vi "GUI - Multi TDMS Files Preview.vi"(5 "error in (no error)":errorcluster, 6 "ReInit All to Default?":bool, 7 "Application Name":string="GenUtil", 9 "State Queue":T1[](array[typedef])=["SC >>> Initialize"]) -> (19 "error out":errorcluster)   [LabVIEW 2020, in "TDMS.lvclass"]
uses:
  TDMS.lvclass
  API/Generic Utilities_class/utils/GenUtil State List.ctl
  <vilib>/Utility/sysdir.llb/System Directory Type.ctl
  <vilib>/Platform/browser.llb/Open URL in Default Browser (path).vi
  API/Generic Utilities_class/Generic Utilities.lvclass
  <vilib>/addons/_AddQ/G#Object/G#Object.lvclass
panel:
  in  "Task":enum32{"Monitor", "Settings"}(tab)
  in  "Select TDMS File":path
  out "group/channel names":string[][](array[string])
  out "value":variant
  out "found":bool
  in  "AppData Folder":bool
  out "State History":string[](array[string])
  out "State Index":i32
  in  "State 1":bool
  in  "Exit":bool
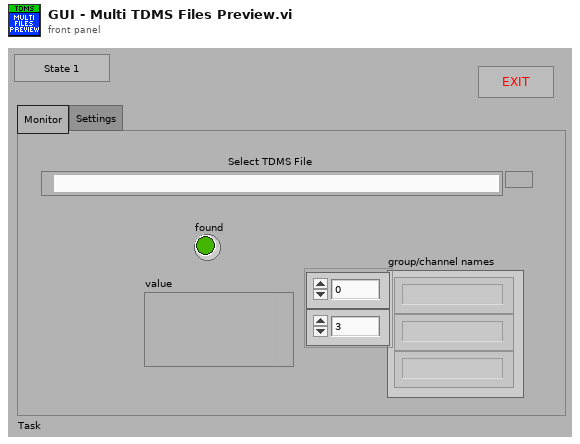
[diagram p1: front panel]
types:
  T1 = typedef "Generic Utilities.lvclass/GenUtil State List.ctl" = string
  T2 = enum32{"Invalid", "Standard", "Closed", "Hidden", "Minimized", "Maximized"}
  T3 = typedef "System Directory Type.ctl" = i32
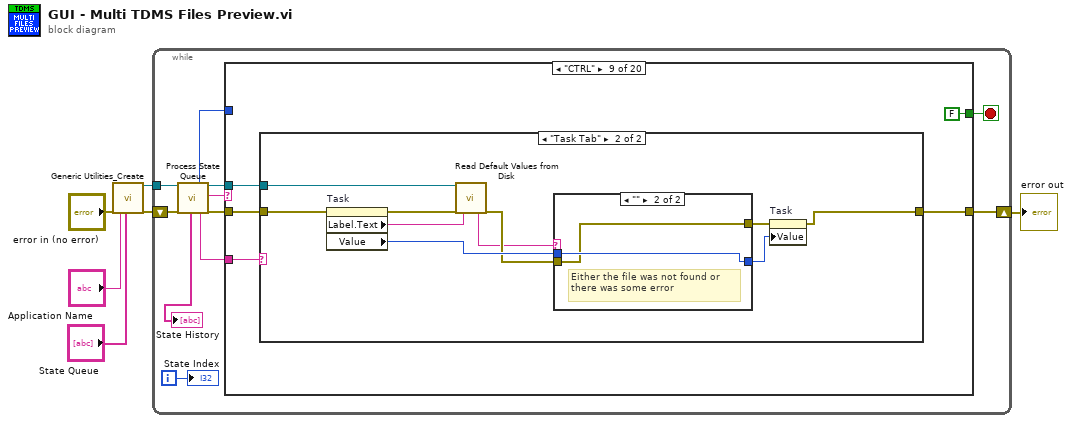
[diagram p0: block diagram]
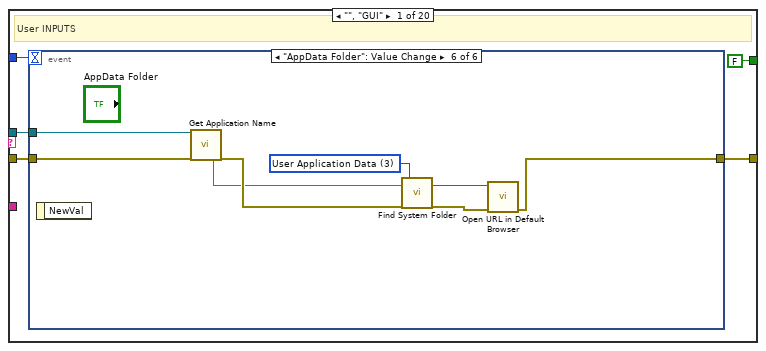
[diagram p2: hidden frame]
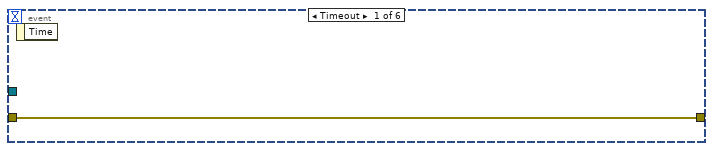
[diagram p3: hidden frame]
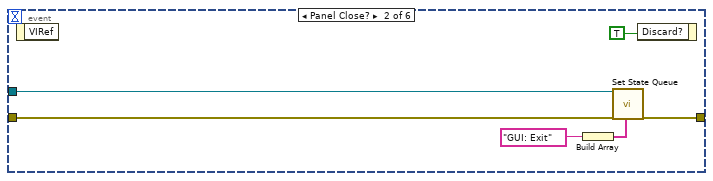
[diagram p4: hidden frame]
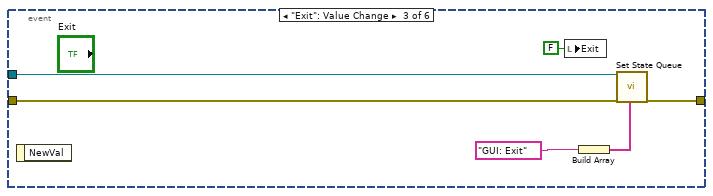
[diagram p5: hidden frame]
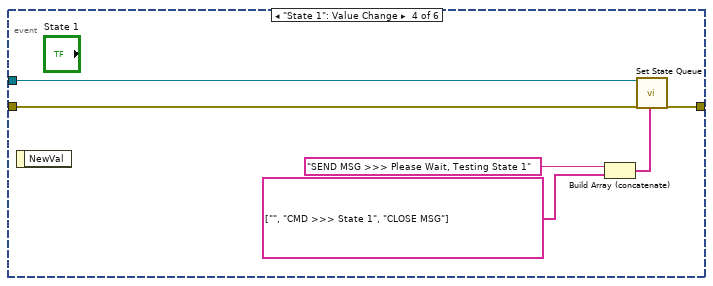
[diagram p6: hidden frame]
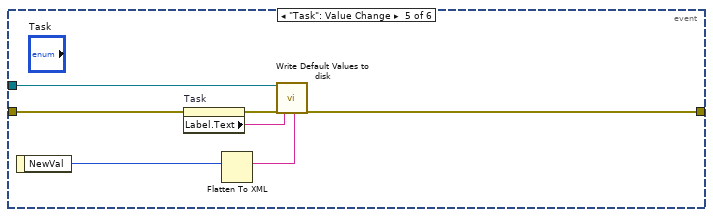
[diagram p7: hidden frame]
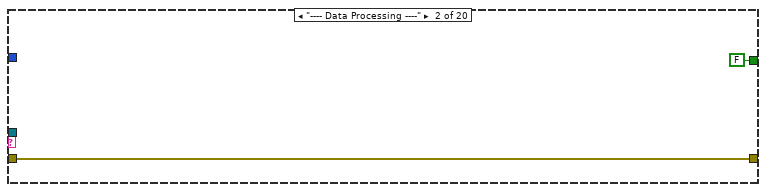
[diagram p8: hidden frame]
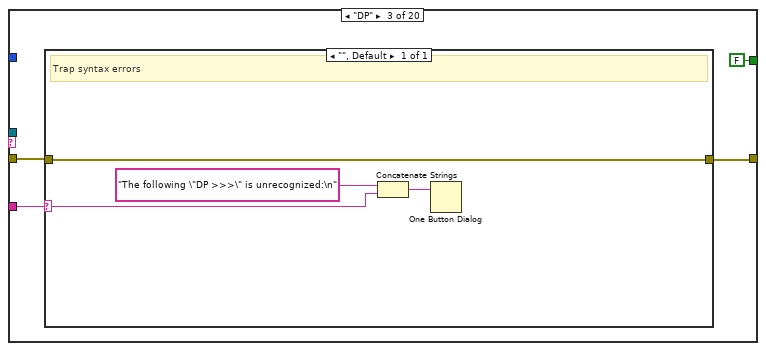
[diagram p9: hidden frame]
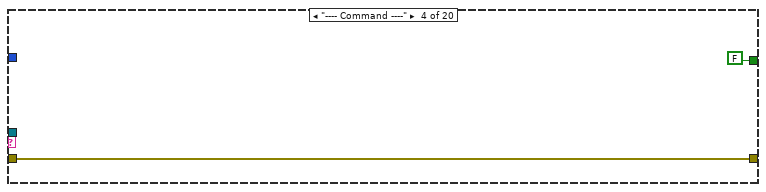
[diagram p10: hidden frame]
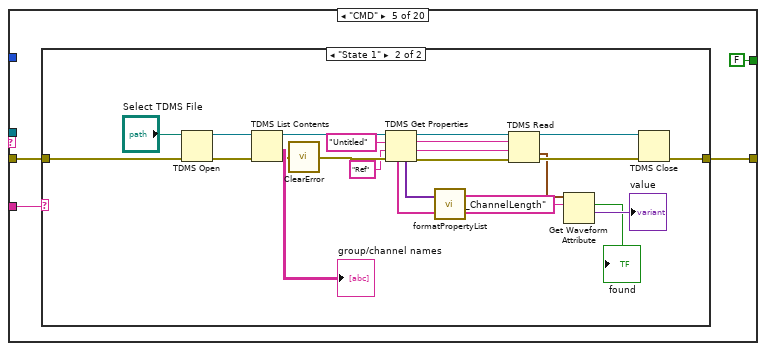
[diagram p11: hidden frame]
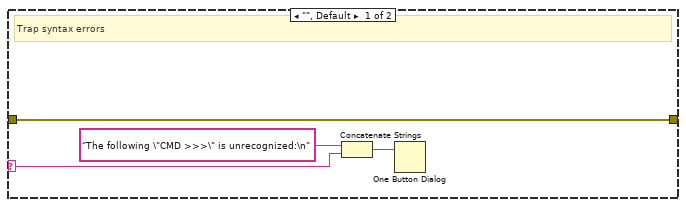
[diagram p12: hidden frame]
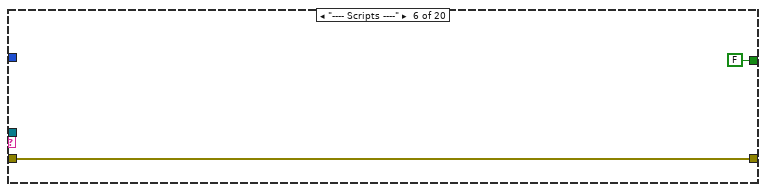
[diagram p13: hidden frame]
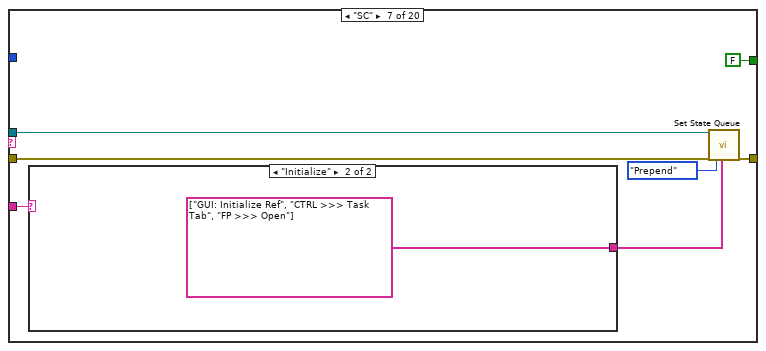
[diagram p14: hidden frame]
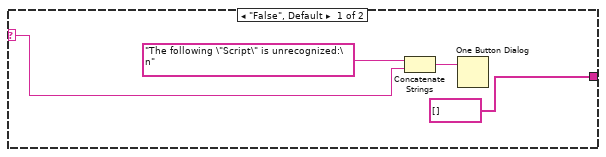
[diagram p15: hidden frame]
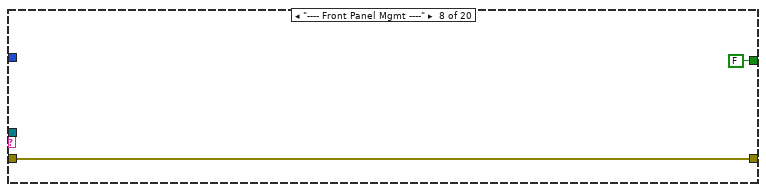
[diagram p16: hidden frame]
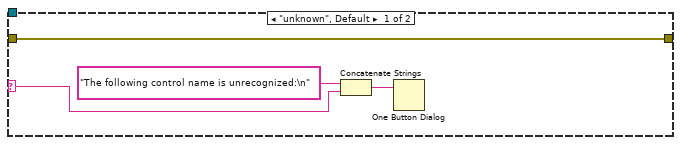
[diagram p17: hidden frame]
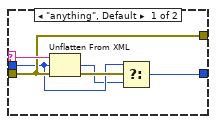
[diagram p18: hidden frame]
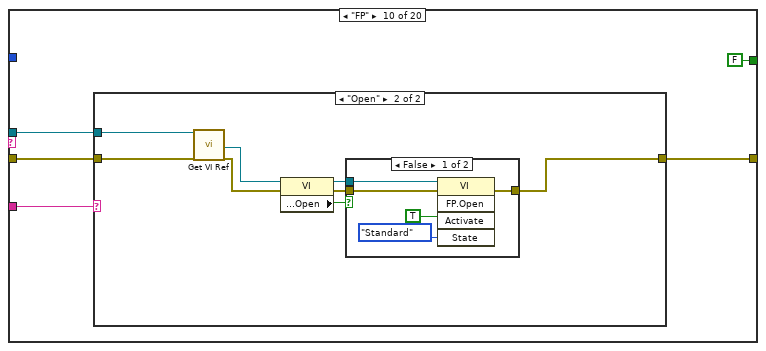
[diagram p19: hidden frame]
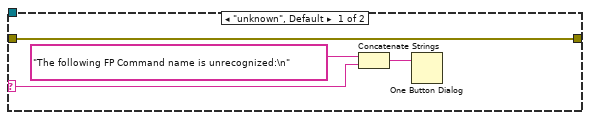
[diagram p20: hidden frame]
diagram:
  n1 = call "Generic Utilities_Create.vi"("error in (no error)"="error in (no error)", "Application Name"="Application Name", "State Queue"="State Queue") -> ("reference out"=w6:refnum<class "Generic Utilities.lvclass">, "error out"=w5:errorcluster)  [unwired: 15 in]
  n2 = while {
    shift-right: [w9] -> w1
    shift-left: w5 -> [w14]
    tunnel: w6 -> [w15]
    i -> [w16]
    stop <- w17 stop-if-true
    n3 = call "Process State Queue.vi"("reference in"=w15, "error in (no error)"=w14) -> ("State History"=→"State History":string[], "Timeout"=w13:i32, "State Option"=w8:string, "reference out"=w12:refnum<class "Generic Utilities.lvclass">, "Current State"=w11:string, "error out"=w10:errorcluster)  [unwired: 10 in, 2 out]
    n4 = case shown="\"CTRL\"" w11 {
      selector: w11 -> [_ _ _ _ _ _ _ _ _ _ _ _ _ _ _ _ w266 _ _ _]
      tunnel: w12 -> [w20 _ _ _ _ _ w107 _ w118 w146 _ w176 w189 w225 w250 _ _ _ _ w276]
      tunnel: [FALSE FALSE FALSE FALSE FALSE FALSE FALSE FALSE FALSE FALSE FALSE FALSE TRUE FALSE FALSE FALSE FALSE FALSE FALSE TRUE] -> w17
      tunnel: w13 -> [w21 _ _ _ _ _ _ _ _ _ _ _ _ _ _ _ _ _ _ _]
      tunnel: w8 -> [_ _ w61 _ w71 _ w103 _ w119 w143 _ _ _ w234 _ _ _ _ _ _]
      tunnel: w10 -> [w19 w57 w60 w67 w69 w100 w106 w114 w116 w145 w166 w172 w186 w224 w251 w262 w264 w269 w272 w275]
      tunnel: [w18 w57 w59 w67 w70 w100 w105 w114 w117 w144 w166 w173 w185 w222 w247 w262 w264 errorcluster {"status"=FALSE, "code"=0, "source"=""} ("error out") w272 w274] -> w9
      frame "", "GUI" {
        # "User INPUTS"
        n5 = event shown="[5] \"AppData Folder\": Value Change" {
          selector: _ -> [_ _ _ _ _ _]
          dyn-events: _ -> [_ _ _ _ _ _]
          timeout: w21 -> [_ _ _ _ _ _]
          tunnel: w20 -> [_ w28 w34 w40 w47 w55]
          tunnel: w19 -> [w23 w27 w32 w39 w44 w54]
          tunnel: [w23 w26 w33 w41 w42 w49] -> w18
          event Timeout {
            n6 = event-data() -> ()  [unwired: 1 in, 1 out]
          }
          event Panel Close? {
            n7 = event-data() -> ()  [unwired: 1 in, 1 out]
            n8 = Build Array(T1 "GUI: Exit" ("State List")) -> (w25:T1[])
            n9 = call "Set State Queue.vi"("reference in"=w28, "error in (no error)"=w27, "State Queue"=w25) -> ("error out"=w26:errorcluster)  [unwired: 15 in, 1 out]
            n10 = event-data("Discard?"=TRUE) -> ()  [unwired: 1 in, 1 out]
          }
          event "Exit": Value Change {
            n11 = event-data() -> ()  [unwired: 1 in, 1 out]
            n12 = local write "Exit"(FALSE ("Exit")) -> ()
            n13 = Build Array(T1 "GUI: Exit" ("State List")) -> (w31:T1[])
            n14 = call "Set State Queue.vi"("reference in"=w34, "error in (no error)"=w32, "State Queue"=w31) -> ("error out"=w33:errorcluster)  [unwired: 15 in, 1 out]
          }
          event "State 1": Value Change {
            n15 = event-data() -> ()  [unwired: 1 in, 1 out]
            n16 = Build Array (concatenate)("SEND MSG >>> Please Wait, Testing State 1" ("String"), T1[] ["", "CMD >>> State 1", "CLOSE MSG"] ("State Queue OUT")) -> (w36:T1[])
            n17 = call "Set State Queue.vi"("reference in"=w40, "error in (no error)"=w39, "State Queue"=w36) -> ("error out"=w41:errorcluster)  [unwired: 15 in, 1 out]
          }
          event "Task": Value Change {
            n18 = event-data() -> ("NewVal"=w48:enum32{"Monitor", "Settings"})  [unwired: 1 in]
            n19 = property on="Task" class="TabCtl (strict)"(error in=w44) -> (error out=w43:errorcluster, "Label.Text"=w46:string)  [unwired: 1 in, 1 out]
            n20 = Flatten To XML(6:w48) -> (2:w45:string)
            n21 = call-dynamic "Write Default Values to disk.vi"("reference in"=w47, "error in (no error)"=w43, "Control Label"=w46, "Value (XML String)"=w45) -> ("error out"=w42:errorcluster)  [unwired: 14 in, 1 out]
          }
          event "AppData Folder": Value Change {
            w56 = T3 3 items=["User Home"=0, "User Desktop"=1, "User Documents"=2, "User Application Data"=3, "User Preferences"=4, "User Temporary"=5, "Public Documents"=6, "Public Application Data"=7, "Public Preferences"=8, "Public Cache"=13, "System Core Libraries"=9, "System Installed Libraries"=10, "Application Files"=11, "Boot Volume Root"=12] ("system directory type")
            n22 = event-data() -> ()  [unwired: 1 in, 1 out]
            n23 = call "Get Application Name.vi"("reference in"=w55, "error in (no error)"=w54) -> ("Application Name"=w52:string, "error out"=w53:errorcluster)  [unwired: 15 in, 1 out]
            n24 = call "Find System Folder.vi"("Application Name"=w52, "error in (no error)"=w53, "system directory type"=w56) -> ("System Folder"=w51:path, "error out"=w50:errorcluster)  [unwired: 15 in]
            n25 = call-poly <vilib>:"Open URL in Default Browser.vi"("error in (no error)"=w50, "path"=w51) -> ("error out"=w49:errorcluster)  [unwired: 4 in, 1 out]
          }
        }
      }
      frame "---- Data Processing ----" {
      }
      frame "DP" {
        n26 = case shown="\"\", Default" w61 {
          selector: w61 -> [w64]
          tunnel: [w63] -> w59
          tunnel: w60 -> [w63]
          frame "", Default {
            # "Trap syntax errors"
            n27 = Concatenate Strings("The following \"DP >>>\" is unrecognized:\n", w64) -> (w65:string)
            n28 = One Button Dialog(message=w65) -> ()  [unwired: 1 in, 1 out]
          }
        }
      }
      frame "---- Command ----" {
      }
      frame "CMD" {
        n29 = case shown="\"State 1\"" w71 {
          selector: w71 -> [w74 _]
          tunnel: [w73 w97] -> w70
          tunnel: w69 -> [w73 w98]
          frame "", Default {
            # "Trap syntax errors"
            n30 = Concatenate Strings("The following \"CMD >>>\" is unrecognized:\n", w74) -> (w75:string)
            n31 = One Button Dialog(message=w75) -> ()  [unwired: 1 in, 1 out]
          }
          frame "State 1" {
            n32 = TDMS Open(8:w98, 11:"Select TDMS File") -> (0:w94:errorcluster, 3:w93:refnum<k34>)  [unwired: 5 in]
            n33 = TDMS List Contents(4:w94, 7:w93) -> (0:w77:errorcluster, 1:→"group/channel names":string[][], 3:w92:refnum<k34>)  [unwired: 1 in, 1 out]
            n34 = call <vilib>:"ClearError.vi"("error in (no error)"=w77) -> ("error out"=w91:errorcluster)
            n35 = TDMS Get Properties(8:w91, 9:"Ref" ("channel name"), 10:"Untitled" ("group name"), 11:w92) -> (0:w84:errorcluster, 1:w83:string, 2:w82:string, 3:w87:refnum<k34>, 4:w96:variant[], 6:w95:string[])  [unwired: 2 out]
            n36 = call <vilib>:"formatPropertyList.vi"("property names"=w95, "property values"=w96) -> ()  [unwired: 1 out]
            n37 = TDMS Read(0:w87, 5:w82, 7:w83, 11:w84) -> (4:w86:refnum<k34>, 10:w81:waveform(dbl), 15:w85:errorcluster)  [unwired: 4 in, 3 out]
            n38 = Get Waveform Attribute(6:"NI_ChannelLength" ("name"), 7:w81) -> (1:→"value":variant, 2:→"found":bool)  [unwired: 2 in, 2 out]
            n39 = TDMS Close(8:w85, 11:w86) -> (0:w97:errorcluster)  [unwired: 1 out]
          }
        }
      }
      frame "---- Scripts ----" {
      }
      frame "SC" {
        n40 = case shown="\"Initialize\"" w103 {
          selector: w103 -> [w110 _]
          tunnel: [string[] [] ("State Queue OUT") string[] ["GUI: Initialize Ref", "CTRL >>> Task Tab", "FP >>> Open"] ("State Queue OUT")] -> w104
          frame "False", Default {
            n41 = Concatenate Strings("The following \"Script\" is unrecognized:\n", w110) -> (w111:string)
            n42 = One Button Dialog(message=w111) -> ()  [unwired: 1 in, 1 out]
          }
          frame "Initialize" {
          }
        }
        n43 = call "Set State Queue.vi"("reference in"=w107, "error in (no error)"=w106, "State Queue Options"=enum16{"Replace", "Append", "Prepend"}."Prepend", "State Queue"=w104) -> ("error out"=w105:errorcluster)  [unwired: 14 in, 1 out]
      }
      frame "---- Front Panel Mgmt ----" {
      }
      frame "CTRL" {
        n44 = case shown="\"Task Tab\"" w119 {
          selector: w119 -> [w123 _]
          tunnel: w118 -> [_ w131]
          tunnel: [w121 w126] -> w117
          tunnel: w116 -> [w121 w129]
          frame "unknown", Default {
            n45 = Concatenate Strings("The following control name is unrecognized:\n", w123) -> (w122:string)
            n46 = One Button Dialog(message=w122) -> ()  [unwired: 1 in, 1 out]
          }
          frame "Task Tab" {
            n47 = property on="Task" class="TabCtl (strict)"(error in=w129) -> (error out=w130:errorcluster, "Label.Text"=w128:string, "Value"=w133:enum32{"Monitor", "Settings"})  [unwired: 1 in, 1 out]
            n48 = call-dynamic "Read Default Values from Disk.vi"("reference in"=w131, "error in (no error)"=w130, "Control Label"=w128) -> ("Value (XML String)"=w125:string, "error out"=w127:errorcluster)  [unwired: 14 in, 1 out]
            n49 = case shown="\"\"" w125 {
              selector: w125 -> [w140 _]
              tunnel: [w135 w142] -> w134
              tunnel: w133 -> [w137 w142]
              tunnel: w127 -> [w138 w141]
              tunnel: [w138 w141] -> w132
              frame "anything", Default {
                n50 = Unflatten From XML(xml string=w140, type=w137, error in (no error)=w138) -> (value=w136:enum32{"Monitor", "Settings"}, error out=w139:errorcluster)
                n51 = Select(t=w137, s=w139, f=w136) -> (s? t:f=w135:enum32{"Monitor", "Settings"})
              }
              frame "" {
                # "Either the file was not found or there was some error"
              }
            }
            n52 = property on="Task" class="TabCtl (strict)"(error in=w132, "Value"=w134) -> (error out=w126:errorcluster)  [unwired: 1 in, 1 out]
          }
        }
      }
      frame "FP" {
        n53 = case shown="\"Open\"" w143 {
          selector: w143 -> [w148 _]
          tunnel: w146 -> [_ w156]
          tunnel: w145 -> [w149 w155]
          tunnel: [w149 w152] -> w144
          frame "unknown", Default {
            n54 = Concatenate Strings("The following FP Command name is unrecognized:\n", w148) -> (w150:string)
            n55 = One Button Dialog(message=w150) -> ()  [unwired: 1 in, 1 out]
          }
          frame "Open" {
            n56 = call-dynamic "Get VI Ref.vi"("reference in"=w156, "error in (no error)"=w155) -> ("GUI VI Ref"=w153:refnum<vi>, "error out"=w154:errorcluster)  [unwired: 14 in, 2 out]
            n57 = property class="VI"(reference=w153, error in=w154) -> (reference out=w158:refnum<vi>, error out=w159:errorcluster, "Front Panel.Open"=w157:bool)
            n58 = case shown="False" w157 {
              tunnel: [w162 w165] -> w152
              tunnel: w159 -> [w161 w165]
              tunnel: w158 -> [w160 _]
              frame False {
                n59 = invoke class="VI" method="FP.Open"(reference=w160, error in=w161, "Activate"=TRUE, "State"=T2."Standard") -> (error out=w162:errorcluster)  [unwired: 1 in, 4 out]
              }
              frame True {
              }
            }
          }
        }
      }
      frame "---- GUI Functions ----" {
      }
      frame "GUI: Initialize Ref" {
        n60 = control-ref of="GUI Reference"() -> (w171:refnum<vi>)
        n61 = call "Set VI Ref.vi"("reference in"=w176, "error in (no error)"=w172, "ReInit All to Default?"="ReInit All to Default?", "GUI VI Ref"=w171) -> ("reference out"=w175:refnum<class "Generic Utilities.lvclass">, "error out"=w170:errorcluster)  [unwired: 14 in]
        n62 = call "Set Close Panel (Yes or No).vi"("reference in"=w175, "error in (no error)"=w170) -> ("reference out"=w174:refnum<class "Generic Utilities.lvclass">, "error out"=w169:errorcluster)  [unwired: 16 in]
        n63 = call "Set Message Window Ref.vi"("reference in"=w174, "error in (no error)"=w169) -> ("error out"=w173:errorcluster)  [unwired: 16 in, 1 out]
      }
      frame "GUI: Exit" {
        n64 = call-dynamic "Get Message Window Ref.vi"("reference in"=w189, "error in (no error)"=w186) -> ("reference out"=w188:refnum<class "Generic Utilities.lvclass">, "Msg Win Ref"=w184:refnum<vi>, "error out"=w187:errorcluster)  [unwired: 15 in]
        n65 = call-dynamic "Get VI Ref.vi"("reference in"=w188, "error in (no error)"=w187) -> ("reference out"=w192:refnum<class "Generic Utilities.lvclass">, "GUI VI Ref"=w190:refnum<vi>, "error out"=w191:errorcluster)  [unwired: 14 in, 1 out]
        n66 = call-dynamic "Get Close Panel (Yes or No).vi"("reference in"=w192, "error in (no error)"=w191) -> ("Close Panel?"=w193:bool, "reference out"=w182:refnum<class "Generic Utilities.lvclass">, "error out"=w183:errorcluster)  [unwired: 15 in]
        n67 = call-dynamic "Get OBJ NOT RefNum.vi"("reference in"=w182, "error in (no error)"=w183) -> ("OBJ not a refnum?"=w181:bool, "reference out"=w180:refnum<class "Generic Utilities.lvclass">, "error out"=w179:errorcluster)  [unwired: 15 in]
        n68 = case shown="True" w181 {
          tunnel: [w198 w201] -> w178
          tunnel: w180 -> [_ w200]
          tunnel: w179 -> [w198 w199]
          frame False {
            # "The OBJ already exist, indicating this is a dialog box or sub-vi so do NOT destroy the original OBJ."
          }
          frame True {
            # "New OBJ was created, so it needs to be deleted."
            n69 = call-dynamic "Destroy.vi"("reference in"=w200, "error in (no error)"=w199) -> ("error out"=w202:errorcluster)  [unwired: 16 in, 1 out]
            n70 = disable-structure shown="Disabled" {
              disable-tunnel: w202 -> [w204 w205]
              disable-tunnel: [w203 w205] -> w201
              frame Disabled {
                # "Enable when NEEDED"
                n71 = call <vilib>:"GarbageCollector.vi"("error in (no error)"=w204) -> ("error out"=w203:errorcluster)  [unwired: 16 in, 2 out]
              }
              frame Enabled {
              }
            }
          }
        }
        n72 = Close Reference(reference=w184, error in (no error)=w178) -> (error out=w196:errorcluster)
        n73 = case shown="True" w193 {
          tunnel: w196 -> [w207 w211]
          tunnel: [w207 w210] -> w194
          tunnel: [w206 w209] -> w195
          tunnel: w190 -> [w206 w208]
          frame False {
          }
          frame True {
            n74 = property class="VI"(reference=w208, error in=w211) -> (reference out=w213:refnum<vi>, error out=w212:errorcluster, "Front Panel.Open"=w214:bool)
            n75 = case shown="True" w214 {
              tunnel: [w216 w220] -> w210
              tunnel: w212 -> [w216 w219]
              tunnel: w213 -> [w215 w218]
              tunnel: [w215 w217] -> w209
              frame False {
              }
              frame True {
                n76 = invoke class="VI" method="FP.Close"(reference=w218, error in=w219) -> (reference out=w217:refnum<vi>, error out=w220:errorcluster)  [unwired: 1 in, 1 out]
              }
            }
          }
        }
        n77 = Close Reference(reference=w195, error in (no error)=w194) -> (error out=w185:errorcluster)
      }
      frame "SEND MSG" {
        n78 = call-dynamic "Get Message Window Ref.vi"("reference in"=w225, "error in (no error)"=w224) -> ("Msg Win Ref"=w221:refnum<vi>, "error out"=w223:errorcluster)  [unwired: 15 in, 1 out]
        n79 = property class="VI"(reference=w221, error in=w223) -> (reference out=w227:refnum<vi>, error out=w226:errorcluster, "Front Panel.Open"=w228:bool)
        n80 = case shown="False" w228 {
          tunnel: [w242 w246] -> w230
          tunnel: w226 -> [w237 w246]
          tunnel: w227 -> [w239 w245]
          tunnel: [w241 w245] -> w229
          frame False {
            w240 = FALSE ("Wait Until Done")
            n81 = invoke class="VI" method="Run VI"(reference=w239, error in=w237, "Wait until done"=w240, "Auto Dispose Ref"=w240) -> (reference out=w238:refnum<vi>, error out=w236:errorcluster)  [unwired: 1 in, 3 out]
            n82 = invoke class="VI" method="FP.Open"(reference=w238, error in=w236, "Activate"=TRUE, "State"=T2."Standard") -> (reference out=w241:refnum<vi>, error out=w242:errorcluster)  [unwired: 1 in, 3 out]
          }
          frame True {
          }
        }
        n83 = Concatenate Strings("\r\n", w234) -> (w233:string)
        n84 = invoke class="VI" method="Ctrl Val.Set"(reference=w229, error in=w230, "Control Name"="Message", "Value"=w233) -> (error out=w222:errorcluster)  [unwired: 1 in, 4 out]
      }
      frame "CLOSE MSG" {
        n85 = call-dynamic "Get Message Window Ref.vi"("reference in"=w250, "error in (no error)"=w251) -> ("Msg Win Ref"=w248:refnum<vi>, "error out"=w249:errorcluster)  [unwired: 15 in, 1 out]
        n86 = property class="VI"(reference=w248, error in=w249) -> (reference out=w253:refnum<vi>, error out=w254:errorcluster, "Front Panel.Open"=w252:bool)
        n87 = case shown="True" w252 {
          tunnel: [w256 w257] -> w247
          tunnel: w254 -> [w256 w261]
          tunnel: w253 -> [_ w260]
          frame False {
          }
          frame True {
            n88 = invoke class="VI" method="FP.Close"(reference=w260, error in=w261) -> (reference out=w259:refnum<vi>, error out=w258:errorcluster)  [unwired: 1 in, 1 out]
            n89 = invoke class="VI" method="Abort VI"(reference=w259, error in=w258) -> (error out=w257:errorcluster)  [unwired: 1 in, 2 out]
          }
        }
      }
      frame "---- Miscelleneous ----" {
      }
      frame "unknown", Default {
        n90 = Concatenate Strings("The following state is unrecognized?\n", w266) -> (w265:string)
        n91 = One Button Dialog(message=w265) -> ()  [unwired: 1 in, 1 out]
      }
      frame "Error" {
        n92 = call <vilib>:"General Error Handler.vi"("error in (no error)"=w269) -> ()  [unwired: 10 in, 5 out]
      }
      frame "Next" {
        # "This is an empty case used so the queue does NOT stop if there is an empty string between two valid states!"
      }
      frame "Quit" {
        # "WARNING!, If the state machine crash, then it will also \"Quit\"??"
        # "This is the case used to simply exit when this GUI is used as a SubVI!"
        n93 = call-dynamic "Destroy.vi"("reference in"=w276, "error in (no error)"=w275) -> ("error out"=w274:errorcluster)  [unwired: 16 in, 1 out]
      }
    }
    "State Index" <- w16
  }
  "error out" <- w1
